vi "imgAddEdit.vi"(8 "error in":errorcluster, 11 "Dev in":refnum<class "Device.lvclass">) -> (0 "error out":errorcluster, 1 "Dev löschen":bool, 2 "Abbruch?":bool, 3 "Dev out":refnum<class "Device.lvclass">)   [LabVIEW 2013]
uses:
  classes/Datastructure/Device/Device.lvclass
panel:
  in  "Dev löschen":bool
  in  "Abbrechen":bool
  in  "OK":bool
  in  "Datum letzter Kalibrierung":string
  in  "Seriennummer":string
  in  "Modell":string
  in  "Hersteller":string
  # "Device erstellen / editieren"
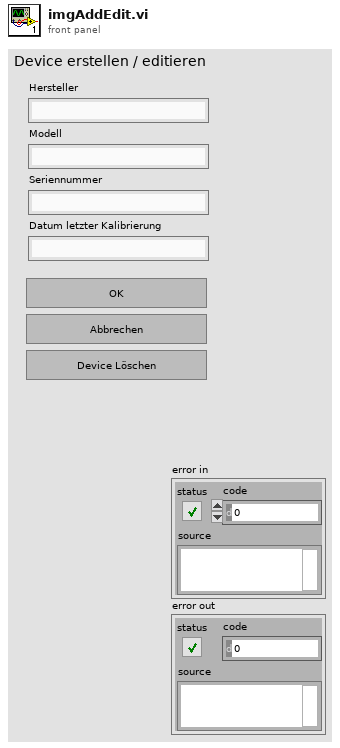
[diagram p1: front panel]
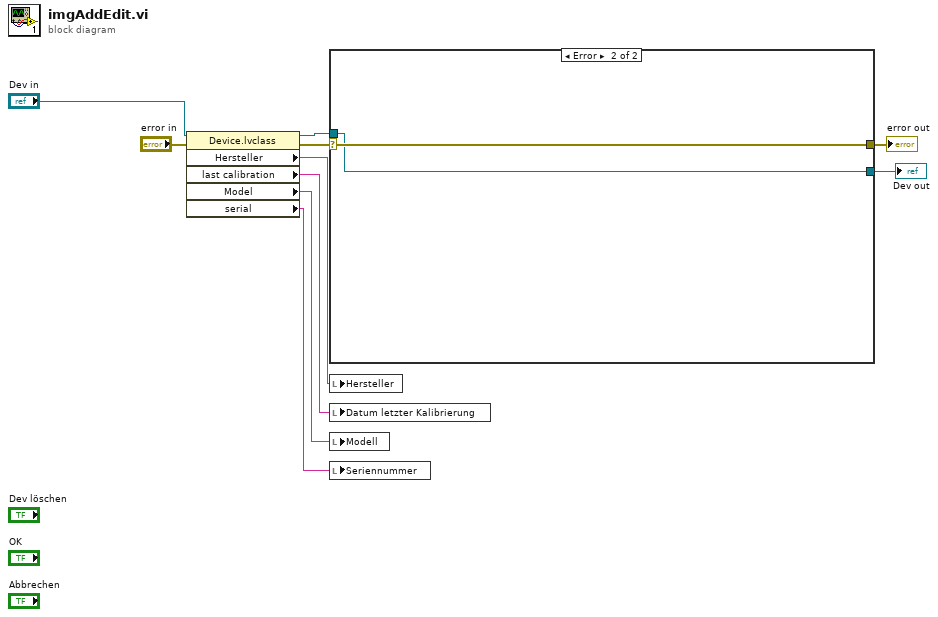
[diagram p0: block diagram]
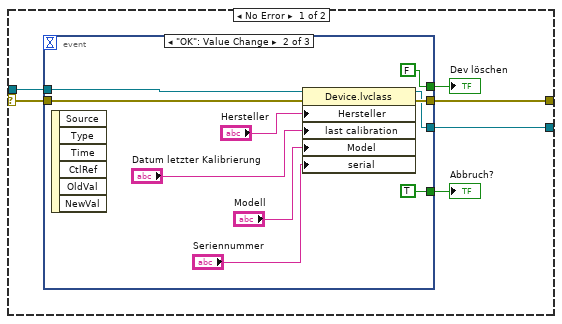
[diagram p2: hidden frame]
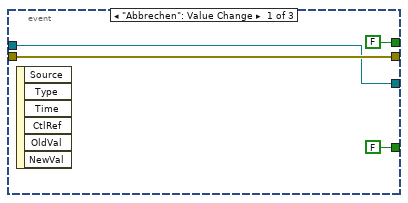
[diagram p3: hidden frame]
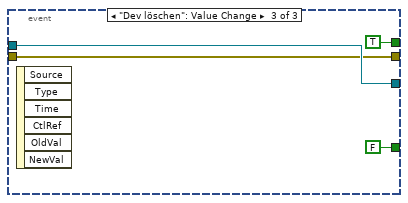
[diagram p4: hidden frame]
diagram:
  n1 = property class="Device.lvclass"(reference="Dev in", error in="error in") -> (reference out=w2:refnum<class "Device.lvclass">, error out=w7:errorcluster, "Hersteller"=w6:string, "last calibration"=w3:string, "Model"=w5:string, "serial"=w4:string)
  n2 = case shown="Error" w7 {
    selector: w7 -> [w14 w36]
    tunnel: [w13 w36] -> w10
    tunnel: [w12 w35] -> w1
    tunnel: w2 -> [w11 w35]
    frame No Error {
      n3 = event shown="[1] \"OK\": Value Change" {
        selector: _ -> [_ _ _]
        dyn-events: _ -> [_ _ _]
        timeout: _ -> [_ _ _]
        tunnel: [FALSE TRUE FALSE] -> w16
        tunnel: [FALSE FALSE TRUE] -> w15
        tunnel: w14 -> [w18 w28 w31]
        tunnel: [w18 w27 w31] -> w13
        tunnel: [w17 w22 w32] -> w12
        tunnel: w11 -> [w17 w21 w32]
        event "Abbrechen": Value Change {
          n4 = event-data() -> ()  [unwired: 1 in, 6 out]
        }
        event "OK": Value Change {
          n5 = event-data() -> ()  [unwired: 1 in, 6 out]
          n6 = property class="Device.lvclass"(reference=w21, error in=w28, "Hersteller"="Hersteller", "last calibration"="Datum letzter Kalibrierung", "Model"="Modell", "serial"="Seriennummer") -> (reference out=w22:refnum<class "Device.lvclass">, error out=w27:errorcluster)
        }
        event "Dev löschen": Value Change {
          n7 = event-data() -> ()  [unwired: 1 in, 6 out]
        }
      }
      "Abbruch?" <- w16
      "Dev löschen" <- w15
    }
    frame Error {
    }
  }
  "error out" <- w10
  "Dev out" <- w1
  n8 = local write "Hersteller"(w6) -> ()
  n9 = local write "Datum letzter Kalibrierung"(w3) -> ()
  n10 = local write "Modell"(w5) -> ()
  n11 = local write "Seriennummer"(w4) -> ()
